vi "HoloCtrlArray.vi"(7 "Action":enum16{"READ", "WRITE"}(ring), 10 "Holo Array In":T1[](array[typedef])) -> (2 "Holo Array Out":T1[](array[typedef]))   [LabVIEW 2018]
uses:
  Controls/Holo Setting.ctl
  Controls/Buttons/Running Button.ctl
  Controls/Zernike Polynominals.ctl
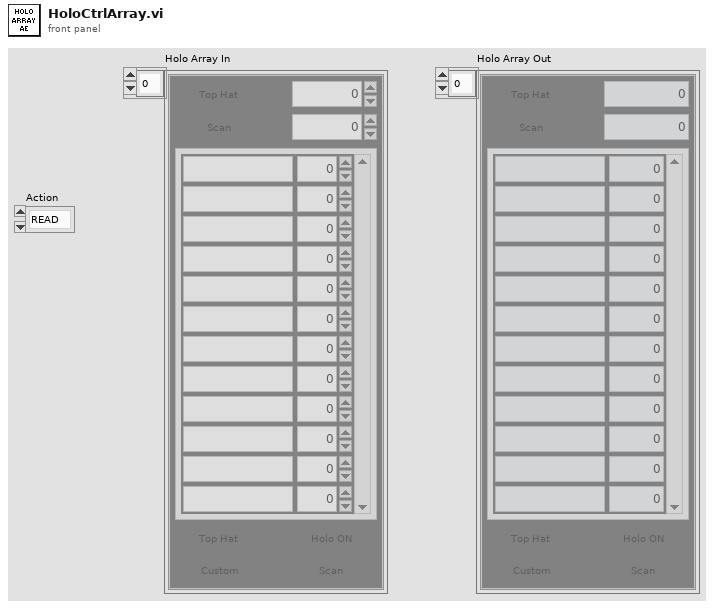
[diagram p1: front panel]
types:
  T1 = typedef "Holo Setting.ctl" = cluster{"Holo On":T2, "Scan":T2, "X":i16, "Y":i16, "Zernike Polynominals":T3, "Top Hat":T2, "Vortex":T2, "Clockwise":T2, "Custom":T2}
  T2 = typedef "Running Button.ctl" = bool
  T3 = typedef "Zernike Polynominals.ctl" = cluster{"Aberration Name":string, "Numeric":dbl}[]
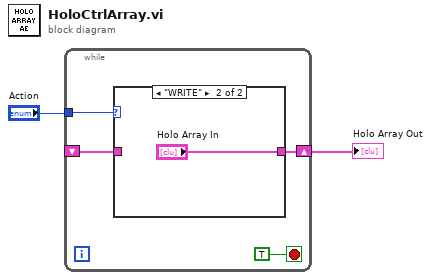
[diagram p0: block diagram]
diagram:
  n1 = while {
    shift-right: [w5] -> w1
    shift-left: _ -> [w4]
    tunnel: "Action" -> [w3]
    stop <- TRUE stop-if-true
    n2 = case shown="\"WRITE\"" w3 {
      tunnel: [w7 "Holo Array In"] -> w5
      tunnel: w4 -> [w7 _]
      frame "READ", Default {
      }
      frame "WRITE" {
      }
    }
  }
  "Holo Array Out" <- w1
